vi "GetSubString.vi"(9 "End Search":string, 10 "Start Search":string, 11 "String In":string) -> (1 "Not Found?":bool, 2 "Match":string, 3 "Following String Out":string)   [LabVIEW 2024]
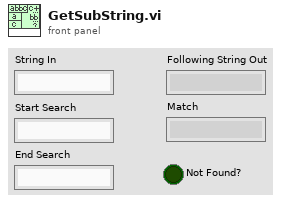
[diagram p1: front panel]
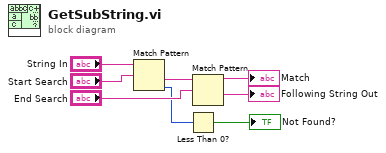
[diagram p0: block diagram]
diagram:
  n1 = Match Pattern(string="String In", regular expression="Start Search") -> (after substring=w7:string, offset past match=w2:i32)  [unwired: 1 in, 2 out]
  n2 = Less Than 0?(x=w2) -> (x < 0?=→"Not Found?":bool)
  n3 = Match Pattern(string=w7, regular expression="End Search") -> (before substring=→"Match":string, after substring=→"Following String Out":string)  [unwired: 1 in, 2 out]
